vi "Get Sender.vi"(11 "TEMPLATE Msg Strategy in":refnum<class "TEMPLATE Msg Strategy.lvclass">) -> (2 "Sender":refnum<class "Sender.lvclass">)   [LabVIEW 2021, in "_Template.lvlib" / "Templates.lvlib" / "TEMPLATE Msg Strategy.lvlib" / "TEMPLATE Msg Strategy.lvclass"]
uses:
  TEMPLATE Msg Strategy.lvclass
  TEMPLATE Msg Strategy.lvclass/TEMPLATE Msg Strategy.ctl
  jettl/jettl/Sender/Sender/Sender.lvclass
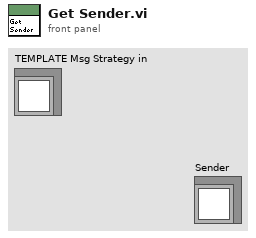
[diagram p1: front panel]
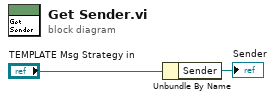
[diagram p0: block diagram]
diagram:
  n1 = Unbundle By Name("TEMPLATE Msg Strategy in") -> ("Sender"=→"Sender":refnum<class "Sender.lvclass">)
